vi "InitializeBtnTabs(SubVI).vi"(8 "error IO":errorcluster, 9 "Switch":refnum<vi>, 10 "Stop acq":refnum<vi>, 11 "Tab Control 2":refnum<vi>) -> (0 "error out":errorcluster)   [LabVIEW 2013, in "main.lvlib"]
uses:
  main.lvlib
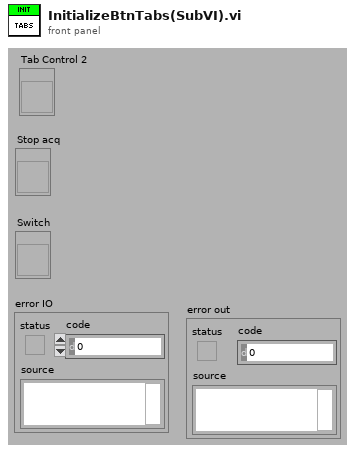
[diagram p1: front panel]
types:
  T1 = enum32{"Profile", "Configuration", "Acquisition", "Data Processing", "View Data"}
  T2 = enum8{"Enabled", "Disabled", "Disabled and Grayed Out"}
  T3 = enum32{"Page Enabled", "Page Disabled", "Page Disabled & Grayed"}
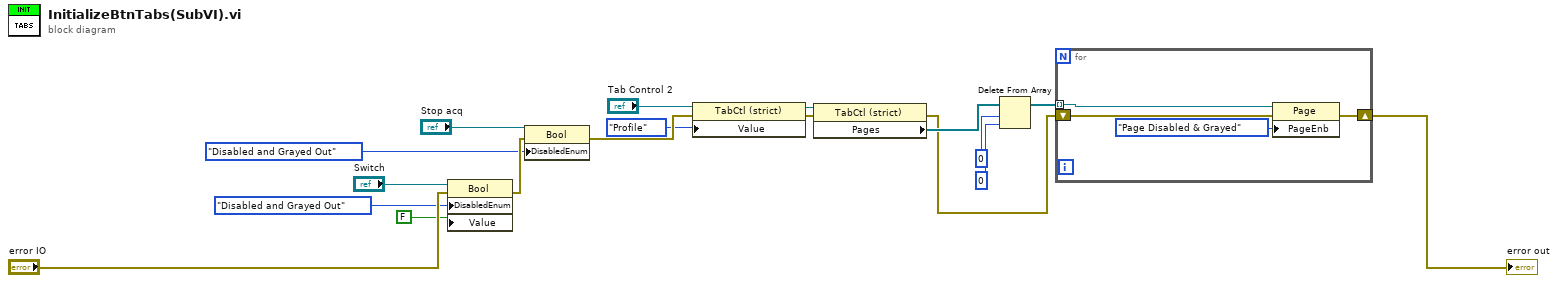
[diagram p0: block diagram]
diagram:
  n1 = property class="Bool"(reference="Switch", error in="error IO", "DisabledEnum"=T2."Disabled and Grayed Out" ("Disabled"), "Value"=FALSE) -> (error out=w15:errorcluster)  [unwired: 1 out]
  n2 = property class="Bool"(reference="Stop acq", error in=w15, "DisabledEnum"=T2."Disabled and Grayed Out" ("Disabled")) -> (error out=w16:errorcluster)  [unwired: 1 out]
  n3 = property class="TabCtl (strict)"(reference="Tab Control 2", error in=w16, "Value"=T1."Profile") -> (reference out=w10:refnum<vi>, error out=w9:errorcluster)
  n4 = property class="TabCtl (strict)"(reference=w10, error in=w9) -> (error out=w6:errorcluster, "Pages"=w8:refnum<vi>[])  [unwired: 1 out]
  n5 = Delete From Array(array=w8, length=0, index=0) -> (array with subset deleted=w7:refnum<vi>[])  [unwired: 1 out]
  n6 = for {
    shift-right: [w22] -> w18
    shift-left: w6 -> [w21]
    tunnel: w7 -> [w19] mode=indexing
    n7 = property class="Page"(reference=w19, error in=w21, "PageEnb"=T3."Page Disabled & Grayed" ("Page Enabled State")) -> (error out=w22:errorcluster)  [unwired: 1 out]
  }
  "error out" <- w18
